vi "UpdateChannelMonitorListbox.vi"(8 "error in (no error)":errorcluster, 10 "Input Channels":T1[](array[typedef]), 11 "Monitored Channels":refnum<vi>) -> (0 "error out":errorcluster)   [LabVIEW 2015, in "Protection and Rolling Counter Addon System Explorer.lvlib"]
uses:
  Protection and Rolling Counter Addon System Explorer.lvlib
  Types/Protection Signal Linked Channels.ctl
  <vilib>/NI Veristand/Custom Device API/Custom Device API.lvlib
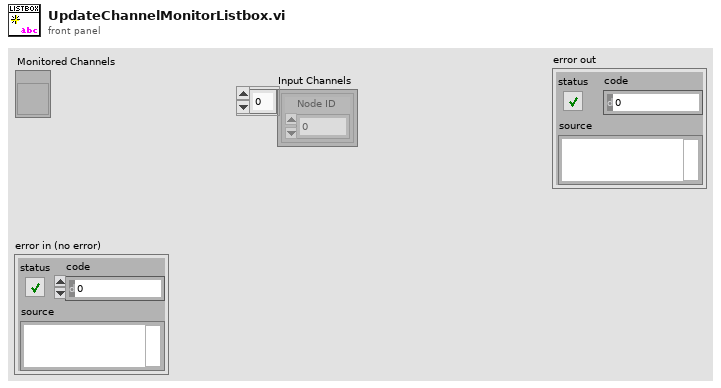
[diagram p1: front panel]
types:
  T1 = typedef "Protection and Rolling Counter Addon System Explorer.lvlib/Protection Signal Linked Channels.ctl" = cluster{"Node ID":u64}
  T2 = typedef "Custom Device API.lvlib/Custom Device Item Info.ctl" = cluster{"Name":string, "Is Channel":bool, "GUID":string, "Is Waveform":bool}
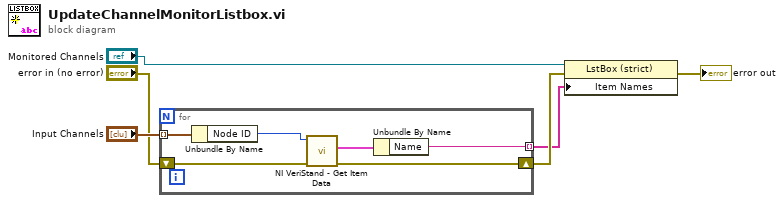
[diagram p0: block diagram]
diagram:
  n1 = for {
    tunnel: "Input Channels" -> [w12] mode=indexing
    shift-right: [w9] -> w2
    shift-left: "error in (no error)" -> [w10]
    tunnel: [w7] -> w1 mode=indexing
    n2 = Unbundle By Name(w12) -> ("Node ID"=w11:u64)
    n3 = call <vilib>:"NI VeriStand - Get Item Data.vi"("error in (no error)"=w10, "Item Ref in"=w11) -> ("error out"=w9:errorcluster, "Item Info"=w8:T2)  [unwired: 6 in, 2 out]
    n4 = Unbundle By Name(w8) -> ("Name"=w7:string)
  }
  n5 = property class="LstBox (strict)"(reference="Monitored Channels", error in=w2, "Item Names"=w1) -> (error out=→"error out":errorcluster)  [unwired: 1 out]
